vi "Get and Write Data..vi"() -> ()   [LabVIEW 2013]
uses:
  DAQ_global.vi
panel:
  out "Datetime":string
  in  "Operator":string
  in  "Путь к файлу протокола":path
  out "Массив данных ()Амплтитуда, частота, Кнли":dbl[][](array[numeric])
  out "Waveform Chart":dbl(graph)
  in  "Задержка, мс":u32
  in  "Число измерений":i32
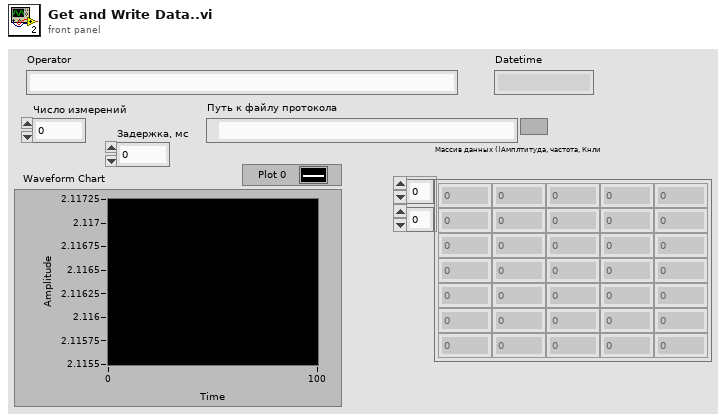
[diagram p1: front panel]
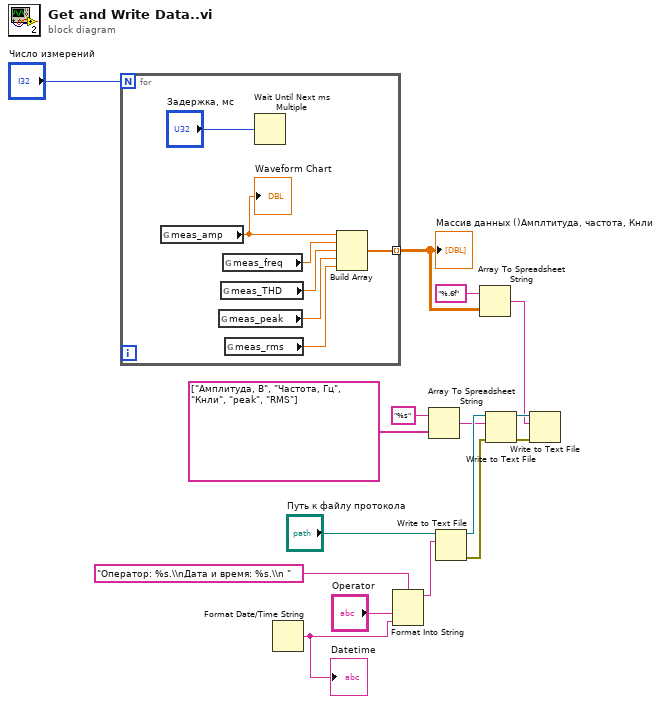
[diagram p0: block diagram]
diagram:
  n1 = for {
    N: "Число измерений" -> [_]
    tunnel: [w19] -> w8 mode=indexing
    n2 = global read "DAQ_global.vi" "meas_amp"() -> (w21:dbl)
    "Waveform Chart" <- w21
    n3 = global read "DAQ_global.vi" "meas_peak"() -> (w18:dbl)
    n4 = global read "DAQ_global.vi" "meas_THD"() -> (w23:dbl)
    n5 = global read "DAQ_global.vi" "meas_freq"() -> (w22:dbl)
    n6 = global read "DAQ_global.vi" "meas_rms"() -> (w17:dbl)
    n7 = Wait Until Next ms Multiple(millisecond multiple="Задержка, мс") -> ()  [unwired: 1 out]
    n8 = Build Array(w21, w22, w23, w18, w17) -> (w19:dbl[])
  }
  "Массив данных ()Амплтитуда, частота, Кнли" <- w8
  n9 = Format Date/Time String() -> (date/time string=w14:string)  [unwired: 3 in]
  "Datetime" <- w14
  n10 = Format Into String(format string="Оператор: %s.\\nДата и время: %s.\\n ", "Operator", w14) -> (resulting string=w7:string)  [unwired: 2 in, 1 out]
  n11 = Array To Spreadsheet String(array=string[] ["Амплитуда, В", "Частота, Гц", "Кнли", "peak", "RMS"], 3:"%s" ("format string")) -> (spreadsheet string=w3:string)  [unwired: 1 in]
  n12 = Write to Text File(file (use dialog)="Путь к файлу протокола", text=w7) -> (refnum out=w5:refnum<file>, error out=w12:errorcluster)  [unwired: 2 in, 1 out]
  n13 = Array To Spreadsheet String(array=w8, 3:"%.6f" ("format string")) -> (spreadsheet string=w2:string)  [unwired: 1 in]
  n14 = Write to Text File(file (use dialog)=w5, text=w3, error in=w12) -> (refnum out=w4:refnum<file>, error out=w11:errorcluster)  [unwired: 1 in, 1 out]
  n15 = Write to Text File(file (use dialog)=w4, text=w2, error in=w11) -> ()  [unwired: 1 in, 3 out]
